vi "State data Look up boolean key.vi"(6 "Error on not found (T)":bool=TRUE, 7 "Key [string/enum]":variant, 8 "error in (no error)":errorcluster, 10 "Value if not found (F)":bool, 11 "Fiber Auto Collimation state data in":refnum<class "Fiber Auto Collimation state data.lvclass">) -> (0 "error out":errorcluster, 1 "Boolean Key found":bool, 2 "Boolean Key Value":bool, 3 "Fiber Auto Collimation state data out":refnum<class "Fiber Auto Collimation state data.lvclass">)   [LabVIEW 2018, in "Fiber Auto Collimation state data.lvclass"]
doc: "Serial number of the Device Under Test."
uses:
  Fiber Auto Collimation state data.lvclass
  Fiber Auto Collimation state data.lvclass/Fiber Auto Collimation state data.ctl
  <userlib>/Recipe/Test Recipe classes/Test Recipe.lvclass
  C:/Program Files (x86)/National Instruments/LabVIEW 2018/user.lib/Recipe/nLight Recipe/nLight Recipe.lvclass
  <userlib>/Recipe/nLight Recipe/nLight Recipe.lvclass
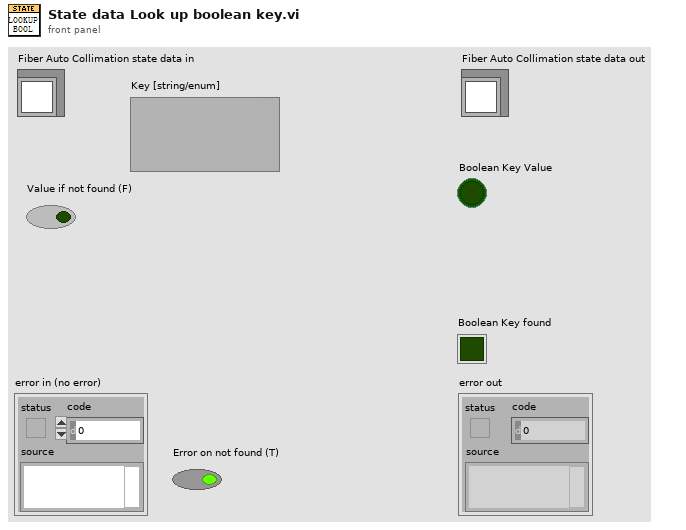
[diagram p1: front panel]
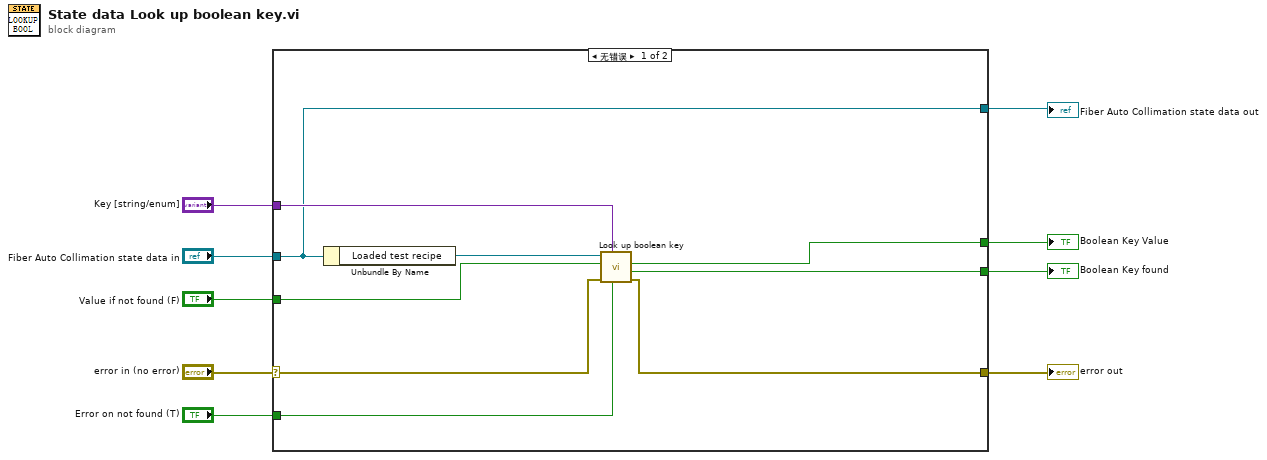
[diagram p0: block diagram]
diagram:
  n1 = case shown="无错误" "error in (no error)" {
    selector: "error in (no error)" -> [w15 w20]
    tunnel: [w12 w20] -> w8
    tunnel: [w16 w19] -> w1
    tunnel: "Fiber Auto Collimation state data in" -> [w16 w19]
    tunnel: "Key [string/enum]" -> [w17 _]
    tunnel: "Error on not found (T)" -> [w13 _]
    tunnel: [w10 _] -> w5
    tunnel: [w11 _] -> w4
    tunnel: "Value if not found (F)" -> [w14 _]
    frame No Error {
      n2 = Unbundle By Name(w16) -> ("Loaded test recipe"=w18:refnum<class "Test Recipe.lvclass">)
      n3 = call <userlib>:"Look up boolean key.vi"("Error on not found (T)"=w13, "Key [string/enum]"=w17, "error in (no error)"=w15, "Value if not found (F)"=w14, "nLight Recipe in"=w18) -> ("error out"=w12:errorcluster, "Boolean Key found"=w11:bool, "Boolean Key Value"=w10:bool)  [unwired: 3 in, 1 out]
    }
    frame Error {
    }
  }
  "Fiber Auto Collimation state data out" <- w1
  "error out" <- w8
  "Boolean Key found" <- w4
  "Boolean Key Value" <- w5
